vi "Math Lookup.vi"() -> ()   [LabVIEW 2014]
doc: "This example shows how to apply a lookup table to an image. Lookup table (LUT) transformations are basic mathematical functions that can be used to improve the contrast and brightness of an image by modifying the intensity dynamics of regions with poor contrast. The LUT can also be used to highlight details in areas containing significant information. In NI Vision, apart from the predefined functions that can be used through the IMAQ MathLookup VI, you can also apply your own lookup tables using the IMAQ UserLookup VI."
uses:
  <vilib>/vision/NI_Vision_Development_Module.lvlib
panel:
  in  "Stop Button":bool
  in  "Operator":T1(ring)=enum."Square"
  in  "X Value":sgl=1.0 min=0 format="%_6g"
  out "LUT Image":T2(plugin-control) caption="Lut Image"
  out "Image Source":T2(plugin-control)
  # "Overview: Demonstrates how to apply a lookup table to an image.\nRequirements: NI Vision Development Module\nInstructions: Run the VI."
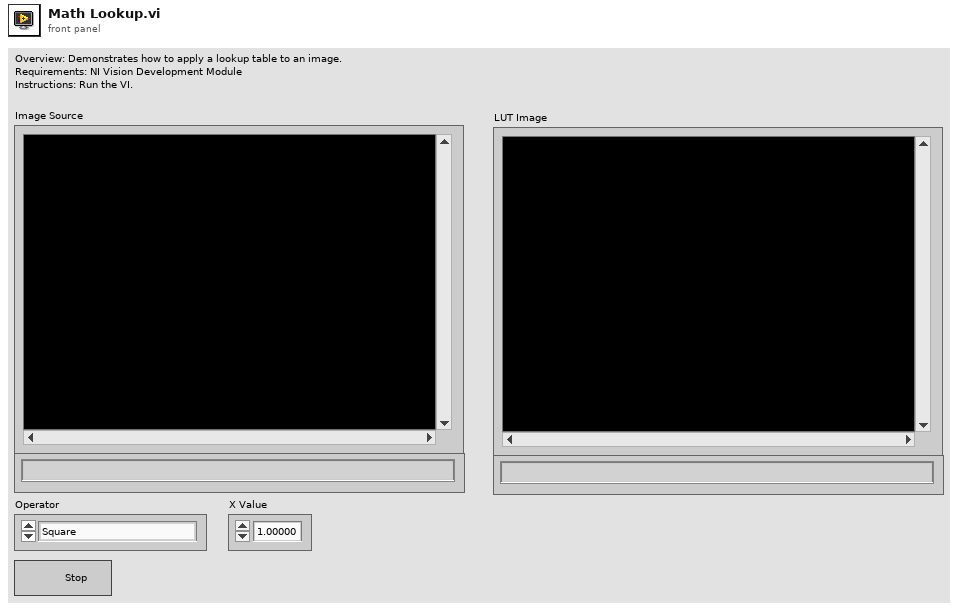
[diagram p1: front panel]
types:
  T1 = enum32{"Linear", "Log", "Exp", "Square", "Square root", "Power X", "Power 1/X"}
  T2 = typedef "IMAQ Image.ctl" = refnum<image>
  T3 = typedef "Image Type" = u32
  T4 = cluster{"X Value":sgl, "Operator":enum32{"Linear", "Log", "Exp", "Square", "Square root", "Power X", "Power 1/X"}}
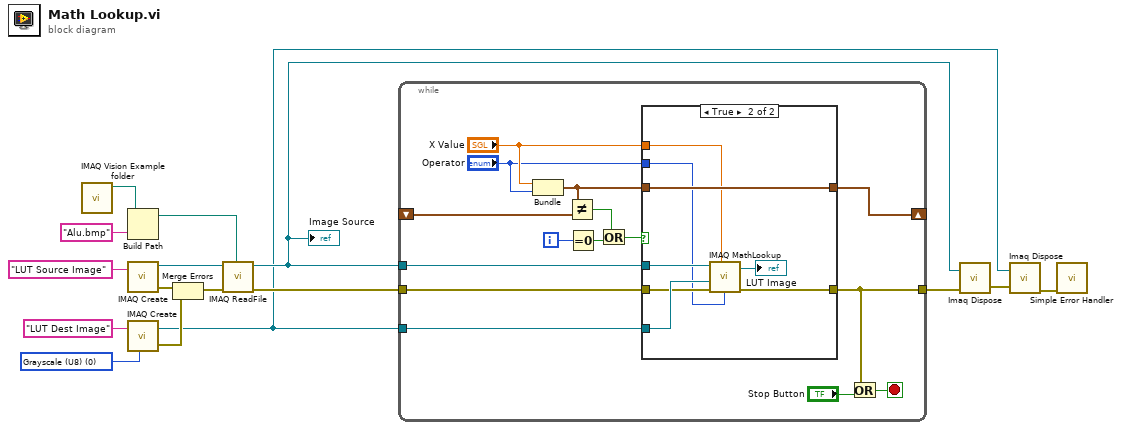
[diagram p0: block diagram]
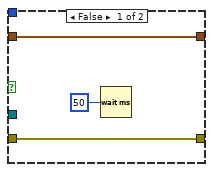
[diagram p2: hidden frame]
diagram:
  w9 = T3 0 items=["Grayscale (U8)", "Grayscale (I16)", "Grayscale (SGL)", "Complex (CSG)", "RGB (U32)", "HSL (U32)", "RGB (U64)", "Grayscale (U16)"] ("Image Type")
  n1 = call "IMAQ Vision Example folder.vi"() -> ("Example Image Path"=w16:path)  [unwired: 11 in]
  n2 = Build Path(base path=w16, name or relative path="Alu.bmp") -> (appended path=w12:path)
  n3 = call "IMAQ Create"("Image Name"="LUT Source Image") -> ("New Image"=w13:T2, "error out"=w6:errorcluster)  [unwired: 4 in]
  n4 = call "IMAQ Create"("Image Name"="LUT Dest Image", "Image Type"=w9) -> ("New Image"=w2:T2, "error out"=w8:errorcluster)  [unwired: 3 in]
  n5 = Merge Errors(w6, w8) -> (w7:errorcluster)
  n6 = call "IMAQ ReadFile"("File Path"=w12, "error in (no error)"=w7, "Image"=w13) -> ("error out"=w5:errorcluster, "Image Out"=w3:T2)  [unwired: 4 in, 3 out]
  "Image Source" <- w3
  n7 = while {
    tunnel: w5 -> [w31]
    tunnel: w3 -> [w30]
    tunnel: w2 -> [w29]
    shift-right: [w28] -> _
    shift-left: _ -> [w27]
    tunnel: [w21] -> w4
    i -> [w26]
    stop <- w20 stop-if-true
    n8 = Bundle("X Value"="X Value", "Operator"="Operator") -> (w17:T4)  [unwired: 1 in]
    n9 = Not Equal?(x=w17, y=w27) -> (x != y?=w25:bool)
    n10 = Equal To 0?(x=w26) -> (x = 0?=w24:bool)
    n11 = Or(x=w25, y=w24) -> (x .or. y?=w23:bool)
    n12 = case shown="True" w23 {
      tunnel: w31 -> [w34 w39]
      tunnel: w30 -> [_ w37]
      tunnel: w17 -> [w33 w42]
      tunnel: w29 -> [_ w41]
      tunnel: [w33 w42] -> w28
      tunnel: [w34 w38] -> w21
      tunnel: "X Value" -> [_ w36]
      tunnel: "Operator" -> [_ w35]
      frame False {
        n13 = Wait (ms)(milliseconds to wait=u32 50) -> ()  [unwired: 1 out]
      }
      frame True {
        n14 = call "IMAQ MathLookup"("Operator"=w35, "X Value"=w36, "error in (no error)"=w39, "Image Dst"=w41, "Image Src"=w37) -> ("error out"=w38:errorcluster, "Image Dst Out"=→"LUT Image":T2)  [unwired: 5 in]
      }
    }
    n15 = Or(x=w21, y="Stop Button") -> (x .or. y?=w20:bool)
  }
  n16 = call "Imaq Dispose"("Image"=w3, "error in (no error)"=w4) -> ("error out"=w1:errorcluster)  [unwired: 4 in]
  n17 = call "Imaq Dispose"("Image"=w2, "error in (no error)"=w1) -> ("error out"=w11:errorcluster)  [unwired: 4 in]
  n18 = call <vilib>:"Simple Error Handler.vi"("error in (no error)"=w11) -> ()  [unwired: 4 in, 5 out]
